vi "example_04_load_from_json.vi"() -> ()   [LabVIEW 2015, in "lv-unit-conversion.lvlib"]
uses:
  lv-unit-conversion.lvlib
panel:
  out "data_set":variant
  out "error":errorcluster
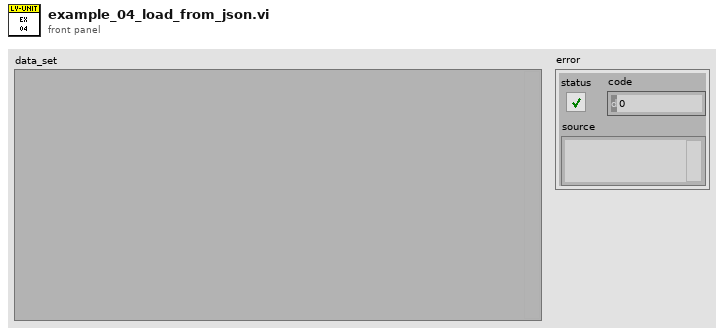
[diagram p1: front panel]
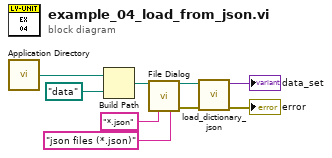
[diagram p0: block diagram]
diagram:
  n1 = call <vilib>:"Application Directory.vi"() -> ("Application Directory"=w9:path)
  n2 = Build Path(base path=w9, name or relative path=path "data" ("Application Directory")) -> (appended path=w5:path)
  n3 = call "File Dialog"("start path"=w5, "pattern (all files)"="*.json", "pattern label"="json files (*.json)") -> ("selected path"=w4:path, "error out"=w3:errorcluster)  [unwired: 9 in, 2 out]
  n4 = call "load_dictionary_json.vi"("error in (no error)"=w3, "json_path"=w4) -> ("error out"=→"error":errorcluster, "unit_dictionary"=→"data_set":variant)  [unwired: 8 in]
